vi "Execute Build.vi"(0 "CLI in":refnum<class "CLI.lvclass">, 5 "All Build Specs":string[](array[string]), 7 "Proj Path":path, 9 "Specs to be built":i32[](array[numeric]), 11 "error in (no error)":errorcluster) -> (4 "CLI out":refnum<class "CLI.lvclass">, 6 "Created Files":path[](array[path]), 15 "error out":errorcluster)   [LabVIEW 2023]
doc: "Execute Build.vi\n----------------------------------------------\nThis SubVI executes the actual build\n\nInputs:\n---------------------\n- All Build Specs : 1DArrayOfString; \n- Proj Path : Path; \n- CLI in : LabVIEW Class Instance; \n- error in (no error) : Cluster; \n- Specs to be built : 1DArrayOfI32; \n\nOutputs:\n---------------------\n- error out : Cluster; \n- CLI out : LabVIEW Class Instance; \n- Created Files : 1DArrayOfPath; \n\n----------------------------------------------\n6/1/2021 nina\nZühlke Engineering AG\nCH-8952 Schlieren\nwww.zuehlke.com"
uses:
  <vilib>/Wiresmith Technology/G CLI/CLI Class/CLI.lvclass
  <vilib>/AppBuilder/AB_API_Simple/Build (path).vi
  <vilib>/AppBuilder/AB_API_Simple/NI_App_Builder_API.lvlib
panel:
  # "Connector Pane"
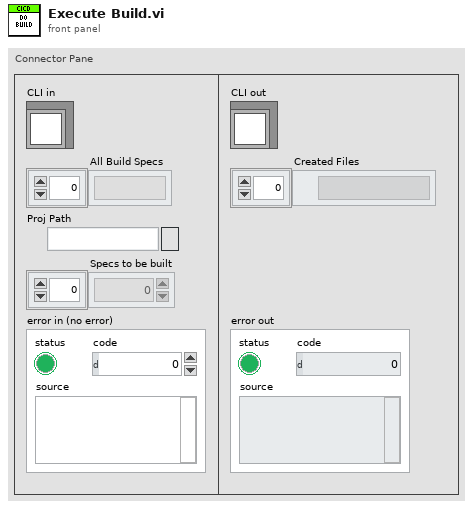
[diagram p1: front panel]
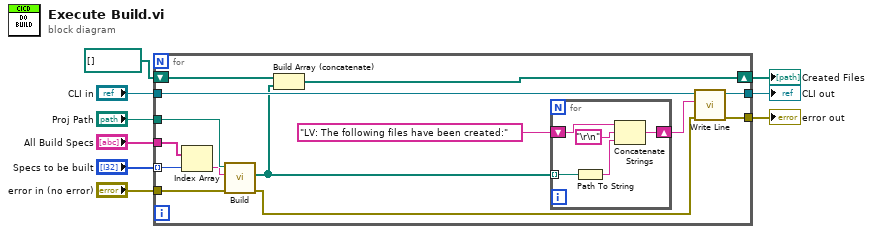
[diagram p0: block diagram]
diagram:
  n1 = for {
    tunnel: "Proj Path" -> [w23]
    tunnel: "Specs to be built" -> [w22] mode=indexing
    tunnel: "CLI in" -> [w21]
    tunnel: [w20] -> w8
    tunnel: "error in (no error)" -> [w16]
    tunnel: [w15] -> w9
    tunnel: "All Build Specs" -> [w14]
    shift-right: [w11] -> w7
    shift-left: path[] [] -> [w10]
    n2 = Index Array(array=w14, index=w22) -> (element=w13:string)
    n3 = call-poly <vilib>:"Build.vi"("error in (no error)"=w16, "Name of build specification (if empty: build all)"=w13, "Path to project"=w23) -> ("error out"=w17:errorcluster, "Generated files"=w12:path[])  [unwired: 7 in]
    n4 = Build Array (concatenate)(w10, w12) -> (w11:path[])
    n5 = for {
      tunnel: w12 -> [w26] mode=indexing
      shift-right: [w24] -> w18
      shift-left: "LV: The following files have been created:" ("Text to Write") -> [w28]
      n6 = Path To String(path=w26) -> (string=w25:string)
      n7 = Concatenate Strings(w28, "\r\n", w25) -> (w24:string)
    }
    n8 = call <vilib>:"Write Line.vi"("error in (no error)"=w17, "Text to Write"=w18, "CLI in"=w21) -> ("error out"=w15:errorcluster, "CLI out"=w20:refnum<class "CLI.lvclass">)  [unwired: 7 in]
  }
  "error out" <- w9
  "CLI out" <- w8
  "Created Files" <- w7
